vi "test_PXI scope fgen sine.vi"() -> ()   [LabVIEW 2023]
uses:
  FGen/FGen PXI/FGen PXI Std Waveform CFG/Std Waveform Action Pams.ctl
  FGen/FGen PXI/FGen PXI Std Waveform CFG/FGen PXI Std Waveform CFG.lvclass
  Scope/Virtual Scopes/Virt Voltage Reader/Virt Voltage Reader.lvclass
  FGen/Virtual FGens/Virt Voltage Generator/Virt Voltage Generator.lvclass
  Scope/Scope PXI/Base CFG/Scope PXI Base CFG.lvclass
  Virtual Instrument Base/Virt Instr Base.lvclass
  <vilib>/Waveform/WDTOps.llb/WDT Number of Waveform Samples DBL.vi
  Measure and Stimulus Subsystems/Measure and Stimulus Subsystems.lvclass
panel:
  out "Sine Gen Chart":waveform(dbl)(graph)
  in  "Std Waveform Pams":T1={"Frequency"=10.0, "Amplitude"=1.0, "DC Offset"=0.0} {"Frequency" format="%#_g Hz"; "Amplitude" format="%#_g V"; "DC Offset" format="%#_g V"}
  out "total samples fetched":i32
  out "#samples fetched":i32[](array[numeric])
  out "Iteration":i32
  in  "Stop":bool
  out "Error Out":errorcluster
  out "Powersensor Scalar":dbl
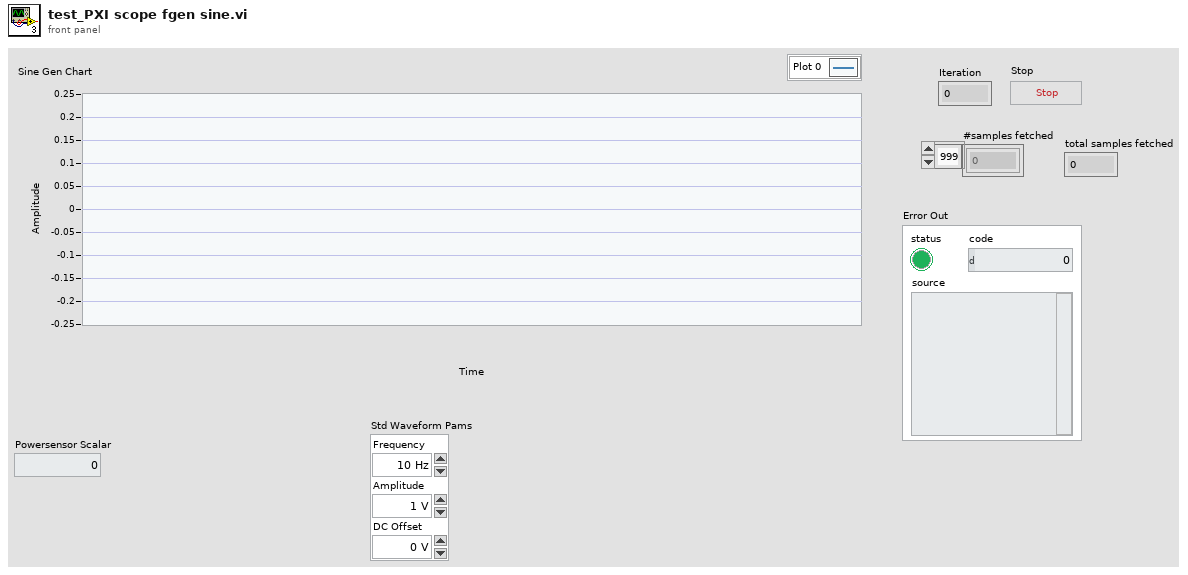
[diagram p1: front panel]
types:
  T1 = typedef "FGen PXI Std Waveform CFG.lvlib/FGen PXI Std Waveform CFG.lvclass/Std Waveform Action Pams.ctl" = cluster{"Frequency":dbl, "Amplitude":dbl, "DC Offset":dbl}
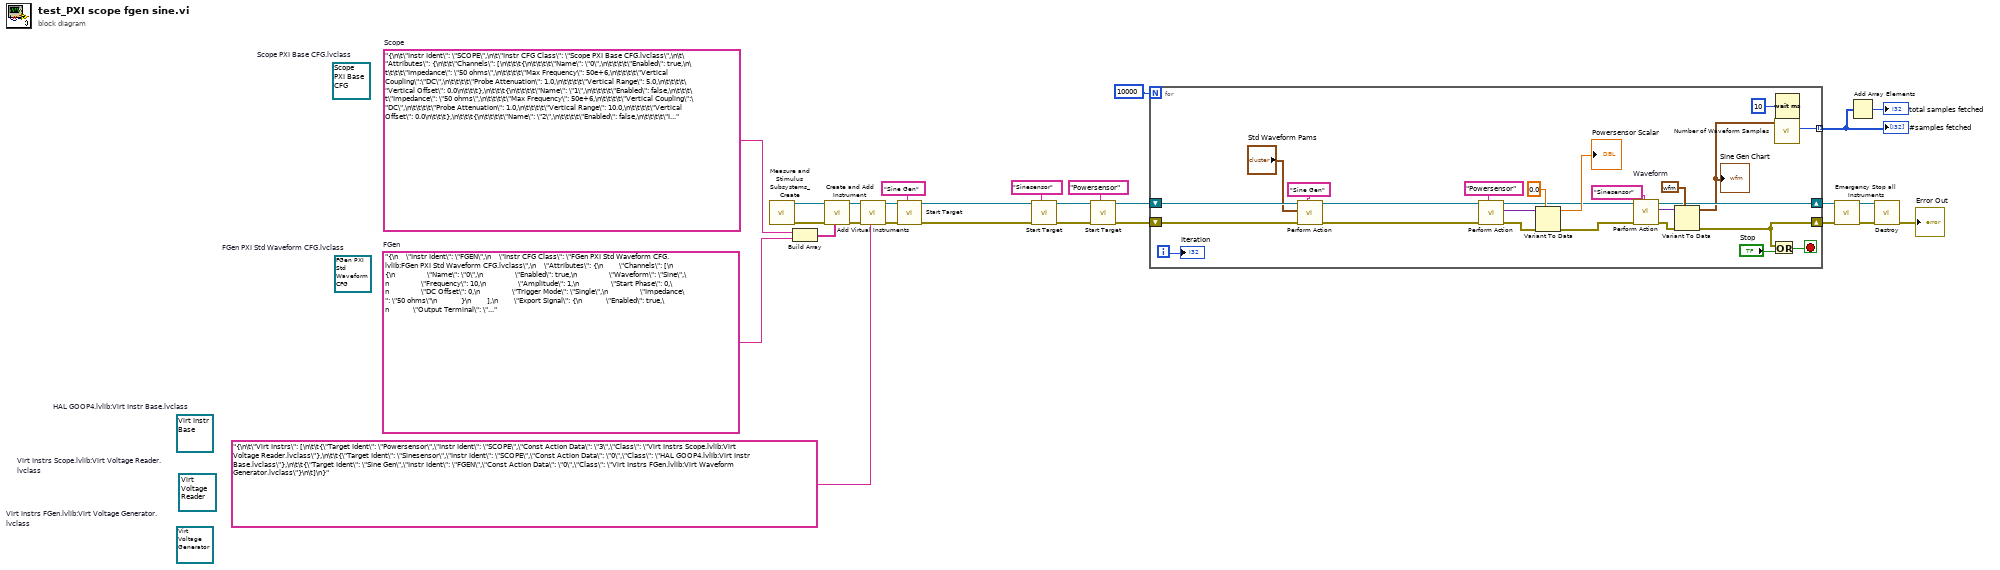
[diagram p0: block diagram]
diagram:
  (unwired) refnum<class "Virt Instr Base.lvclass"> refnum  # HAL GOOP4.lvlib:Virt Instr Base.lvclass
  (unwired) refnum<class "Scope PXI Base CFG.lvclass"> refnum  # Scope PXI Base CFG.lvclass
  (unwired) refnum<class "Virt Voltage Generator.lvclass"> refnum  # Virt Instrs FGen.lvlib:Virt Voltage Generator.lvclass
  (unwired) refnum<class "Virt Voltage Reader.lvclass"> refnum  # Virt Instrs Scope.lvlib:Virt Voltage Reader.lvclass
  (unwired) refnum<class "FGen PXI Std Waveform CFG.lvclass"> refnum  # FGen PXI Std Waveform CFG.lvclass
  w8 = "{\n    \"Instr Ident\": \"FGEN\",\n    \"Instr CFG Class\": \"FGen PXI Std Waveform CFG.lvlib:FGen PXI Std Waveform CFG.lvclass\",\n    \"Attributes\": {\n        \"Channels\": [\n            {\n                \"Name\": \"0\",\n                \"Enabled\": true,\n                \"Waveform\": \"Sine\",\n                \"Frequency\": 10,\n                \"Amplitude\": 1,\n                \"Start Phase\": 0,\n                \"DC Offset\": 0,\n                \"Trigger Mode\": \"Single\",\n                \"Impedance\": \"50 ohms\"\n            }\n        ],\n        \"Export Signal\": {\n            \"Enabled\": true,\n            \"Output Terminal\": \"PFI 0\",\n            \"Signal Identifier\": \"None\",\n            \"Signal\": \"Start Trigger\"\n        },\n        \"Output\": {\n                \"Idle Behavior\": \"Jump To Value\",\n                \"Idle Value\": 0,\n                \"Digital Gain\": 1.0\n        }\n    }\n}"  # FGen
  w16 = "{\n\t\"Instr Ident\": \"SCOPE\",\n\t\"Instr CFG Class\": \"Scope PXI Base CFG.lvclass\",\n\t\"Attributes\": {\n\t\t\"Channels\": [\n\t\t\t{\n\t\t\t\t\"Name\": \"0\",\n\t\t\t\t\"Enabled\": true,\n\t\t\t\t\"Impedance\": \"50 ohms\",\n\t\t\t\t\"Max Frequency\": 50e+6,\n\t\t\t\t\"Vertical Coupling\":\"DC\",\n\t\t\t\t\"Probe Attenuation\": 1.0,\n\t\t\t\t\"Vertical Range\": 5.0,\n\t\t\t\t\"Vertical Offset\": 0.0\n\t\t\t},\n\t\t\t{\n\t\t\t\t\"Name\": \"1\",\n\t\t\t\t\"Enabled\": false,\n\t\t\t\t\"Impedance\": \"50 ohms\",\n\t\t\t\t\"Max Frequency\": 50e+6,\n\t\t\t\t\"Vertical Coupling\":\"DC\",\n\t\t\t\t\"Probe Attenuation\": 1.0,\n\t\t\t\t\"Vertical Range\": 10.0,\n\t\t\t\t\"Vertical Offset\": 0.0\n\t\t\t},\n\t\t\t{\n\t\t\t\t\"Name\": \"2\",\n\t\t\t\t\"Enabled\": false,\n\t\t\t\t\"Impedance\": \"50 ohms\",\n\t\t\t\t\"Max Frequency\": 50e+6,\n\t\t\t\t\"Vertical Coupling\":\"DC\",\n\t\t\t\t\"Probe Attenuation\": 1.0,\n\t\t\t\t\"Vertical Range\": 5.0,\n\t\t\t\t\"Vertical Offset\": 0.0\n\t\t\t},\n\t\t\t{\n\t\t\t\t\"Name\": \"3\",\n\t\t\t\t\"Enabled\": true,\n\t\t\t\t\"Impedance\": \"50 ohms\",\n\t\t\t\t\"Max Frequency\": 50e+6,\n\t\t\t\t\"Vertical Coupling\":\"DC\",\n\t\t\t\t\"Probe Attenuation\": 1.0,\n\t\t\t\t\"Vertical Range\": 1.4,\n\t\t\t\t\"Vertical Offset\": 0.0\n\t\t\t},\n\t\t\t{\n\t\t\t\t\"Name\": \"4\",\n\t\t\t\t\"Enabled\": false,\n\t\t\t\t\"Impedance\": \"50 ohms\",\n\t\t\t\t\"Max Frequency\": 50e+6,\n\t\t\t\t\"Vertical Coupling\":\"DC\",\n\t\t\t\t\"Probe Attenuation\": 1.0,\n\t\t\t\t\"Vertical Range\": 5.0,\n\t\t\t\t\"Vertical Offset\": 0.0\n\t\t\t},\n\t\t\t{\n\t\t\t\t\"Name\": \"5\",\n\t\t\t\t\"Enabled\": false,\n\t\t\t\t\"Impedance\": \"50 ohms\",\n\t\t\t\t\"Max Frequency\": 50e+6,\n\t\t\t\t\"Vertical Coupling\":\"DC\",\n\t\t\t\t\"Probe Attenuation\": 1.0,\n\t\t\t\t\"Vertical Range\": 5.0,\n\t\t\t\t\"Vertical Offset\": 0.0\n\t\t\t},\n\t\t\t{\n\t\t\t\t\"Name\": \"6\",\n\t\t\t\t\"Enabled\": false,\n\t\t\t\t\"Impedance\": \"50 ohms\",\n\t\t\t\t\"Max Frequency\": 50e+6,\n\t\t\t\t\"Vertical Coupling\":\"DC\",\n\t\t\t\t\"Probe Attenuation\": 1.0,\n\t\t\t\t\"Vertical Range\": 5.0,\n\t\t\t\t\"Vertical Offset\": 0.0\n\t\t\t},\n\t\t\t{\n\t\t\t\t\"Name\": \"7\",\n\t\t\t\t\"Enabled\": false,\n\t\t\t\t\"Impedance\": \"50 ohms\",\n\t\t\t\t\"Max Frequency\": 50e+6,\n\t\t\t\t\"Vertical Coupling\":\"DC\",\n\t\t\t\t\"Probe Attenuation\": 1.0,\n\t\t\t\t\"Vertical Range\": 5.0,\n\t\t\t\t\"Vertical Offset\": 0.0\n\t\t\t}\n\t\t],\n\t\t\"Horizontal\": {\n\t\t\t\"Enforce Realtime\": true,\n\t\t\t\"Number of Records\": 1,\n\t\t\t\"Min Sample Rate\": 1e+5,\n\t\t\t\"Reference Position\":10, //percent\n\t\t\t\"Min Record Length\":1e+3\n\t\t},\n\t\t\"Acquire\": {\n\t\t\t\"Type\": \"Normal\",\n\t\t\t\"NumSamples\": 1e+4,\n  \t\"Fetch Relative To\": \"Read Pointer\" \n\t\t},\n\t\t\"Export Signal\": {\n\t\t\t\"Signal Identifier\": \"None\",\n\t\t\t\"Signal\": \"None\",\n\t\t\t\"Output Terminal\": \"None\"\n\t\t},\n\t\t\"Trigger\": {\n\t\t\t\"Type\": \"Software\",\n\t\t\t\"Slope\": \"Positive\",\n\t\t\t\"Source\": \"RTSI 0\",\n\t\t\t\"Holdoff\": 0.0,\n\t\t\t\"Delay\": 0.0\n\t\t}\n\t}\n}"  # Scope
  n1 = call "Measure and Stimulus Subsystems_Create.vi"() -> ("Error Out"=w26:errorcluster, "reference out"=w27:refnum<class "Measure and Stimulus Subsystems.lvclass">)  [unwired: 10 in]
  n2 = Build Array(w16, w8) -> (w15:string[])
  n3 = call "Create and Add Instrument.vi"("Physical Intr Configs"=w15, "Error In"=w26, "reference in"=w27) -> ("Error Out"=w25:errorcluster, "reference out"=w3:refnum<class "Measure and Stimulus Subsystems.lvclass">)  [unwired: 7 in]
  n4 = call "Add Virtual Instruments.vi"("<JSON CFG>"="{\n\t\"Virt Instrs\": [\n\t\t{\"Target Ident\": \"Powersensor\",\"Instr Ident\": \"SCOPE\",\"Const Action Data\": \"3\",\"Class\": \"Virt Instrs Scope.lvlib:Virt Voltage Reader.lvclass\"},\n\t\t{\"Target Ident\": \"Sinesensor\",\"Instr Ident\": \"SCOPE\",\"Const Action Data\": \"0\",\"Class\": \"HAL GOOP4.lvlib:Virt Instr Base.lvclass\"},\n\t\t{\"Target Ident\": \"Sine Gen\",\"Instr Ident\": \"FGEN\",\"Const Action Data\": \"0\",\"Class\": \"Virt Instrs FGen.lvlib:Virt Waveform Generator.lvclass\"}\n\t]\n}", "Error In"=w25, "reference in"=w3) -> ("Error Out"=w4:errorcluster, "reference out"=w2:refnum<class "Measure and Stimulus Subsystems.lvclass">)  [unwired: 7 in]
  n5 = call "Start Target.vi"("Target Ident"="Sine Gen", "Error In"=w4, "reference in"=w2) -> ("Error Out"=w7:errorcluster, "reference out"=w5:refnum<class "Measure and Stimulus Subsystems.lvclass">)  [unwired: 7 in]
  n6 = call "Start Target.vi"("Target Ident"="Sinesensor" ("Target Identifier"), "Error In"=w7, "reference in"=w5) -> ("Error Out"=w18:errorcluster, "reference out"=w11:refnum<class "Measure and Stimulus Subsystems.lvclass">)  [unwired: 7 in]
  n7 = call "Start Target.vi"("Target Ident"="Powersensor", "Error In"=w18, "reference in"=w11) -> ("Error Out"=w12:errorcluster, "reference out"=w10:refnum<class "Measure and Stimulus Subsystems.lvclass">)  [unwired: 7 in]
  n8 = for {
    N: 10000 -> [_]
    shift-right: [w34] -> w20
    shift-left: w12 -> [w50]
    shift-right: [w32] -> w23
    shift-left: w10 -> [w40]
    tunnel: [w41] -> w14 mode=indexing
    i -> [w42]
    stop <- w43 stop-if-true
    w33 = waveform(dbl) {"t0"=timestamp(0 s since 1904-01-01), "dt"=1.0, "Y"=[]}  # Waveform
    n9 = call "Perform Action.vi"("Target Ident"="Sine Gen", "Error In"=w50, "Input"="Std Waveform Pams", "reference in"=w40) -> ("Error Out"=w39:errorcluster, "reference out"=w38:refnum<class "Measure and Stimulus Subsystems.lvclass">)  [unwired: 5 in, 1 out]
    n10 = call "Perform Action.vi"("Target Ident"="Powersensor" ("Target Identifier"), "Error In"=w39, "reference in"=w38) -> ("Error Out"=w51:errorcluster, "Output"=w49:variant, "reference out"=w35:refnum<class "Measure and Stimulus Subsystems.lvclass">)  [unwired: 6 in]
    n11 = Variant To Data(error in=w51, type=0.0, Variant=w49) -> (data=→"Powersensor Scalar":dbl, error out=w44:errorcluster)
    n12 = call "Perform Action.vi"("Target Ident"="Sinesensor", "Error In"=w44, "reference in"=w35) -> ("Error Out"=w30:errorcluster, "Output"=w31:variant, "reference out"=w32:refnum<class "Measure and Stimulus Subsystems.lvclass">)  [unwired: 6 in]
    n13 = Variant To Data(error in=w30, type=w33, Variant=w31) -> (data=w28:waveform(dbl), error out=w34:errorcluster)
    "Sine Gen Chart" <- w28
    n14 = Or(x=w34, y="Stop") -> (x .or. y?=w43:bool)
    n15 = call-poly <vilib>:"Number of Waveform Samples.vi"("waveform in"=w28) -> ("number of samples"=w41:i32)  [unwired: 8 in, 2 out]
    n16 = Wait (ms)(milliseconds to wait=u32 10) -> ()  [unwired: 1 out]
    "Iteration" <- w42
  }
  "#samples fetched" <- w14
  n17 = call "Emergency Stop all Instruments.vi"("Error In"=w20, "reference in"=w23) -> ("Error Out"=w24:errorcluster, "reference out"=w22:refnum<class "Measure and Stimulus Subsystems.lvclass">)  [unwired: 8 in]
  n18 = Add Array Elements(numeric array=w14) -> (sum=→"total samples fetched":i32)
  n19 = call "Destroy.vi"("Error In"=w24, "reference in"=w22) -> ("Error Out"=→"Error Out":errorcluster)  [unwired: 8 in, 1 out]
